vi "Custom Drive Back at angle 119.275.vi"(1 "stop 2":bool, 9 "stop":bool, 10 "Angle":dbl, 11 "RobotDriveDevRef in":T1) -> (2 "i":i32, 3 "RobotDriveDevRef out":T1)   [LabVIEW 2015]
uses:
  <vilib>/Rock Robotics/WPI/RobotDrive/WPI_RobotDriveDevRef.ctl
  <vilib>/Rock Robotics/WPI/MotorControl/WPI_MotorControlDeviceRef.ctl
  <vilib>/Rock Robotics/WPI/MotorControl/WPI_MotorControlType.ctl
  <vilib>/Rock Robotics/SystemInterfaces/DIO/FPGA_DIOPWMChannel.ctl
  <vilib>/Rock Robotics/WPI/PWM/WPI_PWMDeadband.ctl
  <vilib>/Rock Robotics/WPI/CAN/Jaguar/SubVIs/WPI_CANJaguar_ControlMode.ctl
  <vilib>/Rock Robotics/WPI/CAN/TalonSRX/WPI_CANTalonSRX_APIControlMode.ctl
  <vilib>/Rock Robotics/Network Tables/NT Read Number.vi
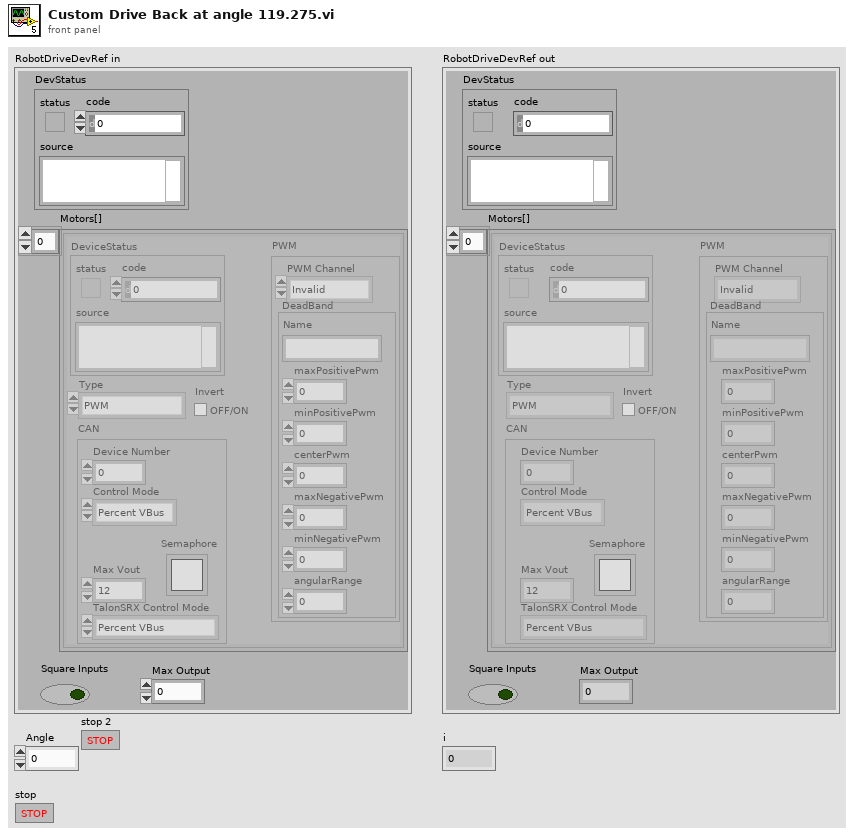
[diagram p1: front panel]
types:
  T1 = typedef "WPI_RobotDriveDevRef.ctl" = cluster{"DevStatus":errorcluster, "Motors[]":T2[], "Square Inputs":bool, "Max Output":dbl}
  T2 = typedef "WPI_MotorControlDeviceRef.ctl" = cluster{"DeviceStatus":errorcluster, "Type":T3, "PWM":cluster{"PWM Channel":T4, "DeadBand":T5}, "CAN":cluster{"Device Number":u8, "Control Mode":T6, "Semaphore":T7, "Max Vout":dbl, "TalonSRX Control Mode":T8}, "Invert":bool}
  T3 = typedef "WPI_MotorControlType.ctl" = enum16{"PWM", "CAN", "CANTalonSRX"}
  T4 = typedef "FPGA_DIOPWMChannel.ctl" = enum8{"PWM 0", "PWM 1", "PWM 2", "PWM 3", "PWM 4", "PWM 5", "PWM 6", "PWM 7", "PWM 8", "PWM 9", "PWM MXP 0", "PWM MXP 1", "PWM MXP 2", "PWM MXP 3", "PWM MXP 4", "PWM MXP 5", "PWM MXP 6", "PWM MXP 7", "PWM MXP 8", "PWM MXP 9", "Invalid"}
  T5 = typedef "WPI_PWMDeadband.ctl" = cluster{"Name":string, "maxPositivePwm":i32, "minPositivePwm":i32, "centerPwm":i32, "maxNegativePwm":i32, "minNegativePwm":i32, "angularRange":u16}
  T6 = typedef "WPI_CANJaguar_ControlMode.ctl" = enum8{"Percent VBus", "Current", "Speed", "Position", "Voltage"}
  T7 = typedef "Semaphore RefNum" = refnum<k1>
  T8 = typedef "WPI_CANTalonSRX_APIControlMode.ctl" = enum8{"Percent VBus", "Speed", "Position", "Slave", "Unchanged / Invalid", "Voltage Compensation", "Current", "Motion Profile"}
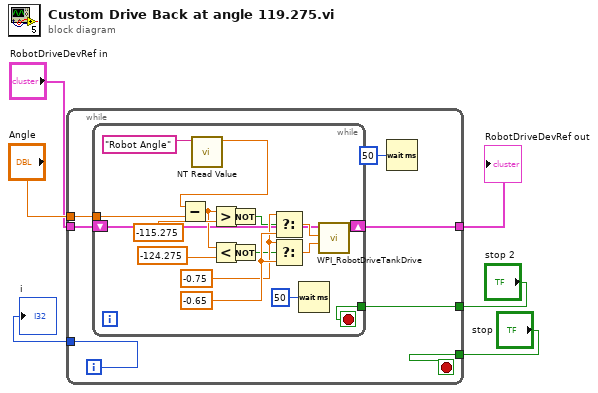
[diagram p0: block diagram]
diagram:
  n1 = while {
    tunnel: "Angle" -> [w13]
    tunnel: "RobotDriveDevRef in" -> [w12]
    tunnel: [w11] -> w4
    tunnel: [w9] -> w3
    tunnel: "stop" -> [w8]
    tunnel: "stop 2" -> [w7]
    i -> [w9]
    stop <- w8 stop-if-true
    n2 = while {
      tunnel: w13 -> [w19]
      shift-right: [w16] -> w11
      shift-left: w12 -> [w17]
      tunnel: w7 -> [w14]
      stop <- w14 stop-if-true
      w29 = -0.65
      w28 = -0.75
      n3 = call-poly <vilib>:"NT Read Value.vi"("Name"="Robot Angle") -> ("Numeric"=w20:dbl)  [unwired: 9 in, 1 out]
      n4 = Subtract(x=w20, y=w19) -> (x-y=w21:dbl)
      n5 = Greater?(x=w21, y=-115.275) -> (0:w24:bool)
      n6 = Less?(x=w21, y=-124.275) -> (x < y?=w25:bool)
      n7 = Not(x=w24) -> (.not. x?=w26:bool)
      n8 = Not(x=w25) -> (.not. x?=w27:bool)
      n9 = Select(t=w28, s=w26, f=w29) -> (s? t:f=w30:dbl)
      n10 = Select(t=w28, s=w27, f=w29) -> (s? t:f=w31:dbl)
      n11 = Wait (ms)(milliseconds to wait=u32 50) -> ()  [unwired: 1 out]
      n12 = call <vilib>:"WPI_RobotDriveTankDrive.vi"("Right axis value"=w31, "Left axis value"=w30, "RobotDriveDevRef"=w17) -> ("RobotDriveDevRef"=w16:T1)  [unwired: 6 in, 2 out]
    }
    n13 = Wait (ms)(milliseconds to wait=u32 50) -> ()  [unwired: 1 out]
  }
  "RobotDriveDevRef out" <- w4
  "i" <- w3
